vi "示例 3.vi"() -> ()   [LabVIEW 2021]
panel:
  out "min":dbl
  out "max":dbl
  in  "b":dbl
  in  "a":dbl
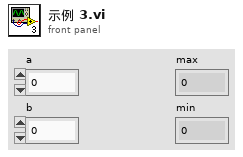
[diagram p1: front panel]
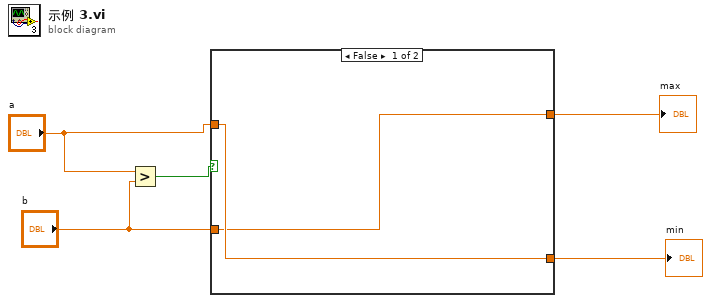
[diagram p0: block diagram]
diagram:
  n1 = Greater?(x="a", y="b") -> (0:w5:bool)
  n2 = case shown="False" w5 {
    tunnel: "a" -> [w7 w9]
    tunnel: "b" -> [w6 w8]
    tunnel: [w6 w9] -> w2
    tunnel: [w7 w8] -> w1
    frame False {
    }
    frame True {
    }
  }
  "max" <- w2
  "min" <- w1
